vi "Move Picture Add Delta.vi"(6 "Delta":cluster{"y":i16, "x":i16}, 7 "Function":enum16{"nop", "point", "rect"}(ring), 9 "index":i32, 10 "Picture In":u8[](array[numeric])) -> (2 "Picture Out":u8[](array[numeric]))   [LabVIEW 2023]
doc: "Wiebe Walstra\nwww.carya.nl"
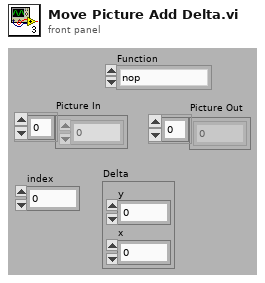
[diagram p1: front panel]
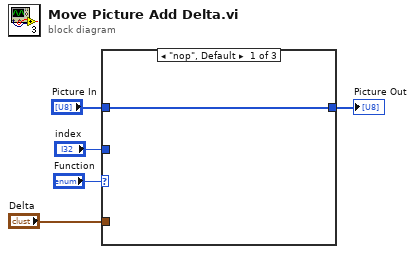
[diagram p0: block diagram]
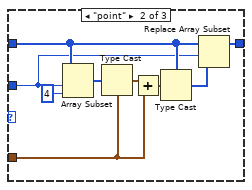
[diagram p2: hidden frame]
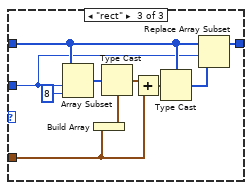
[diagram p3: hidden frame]
diagram:
  n1 = case shown="\"nop\", Default" "Function" {
    tunnel: [w6 w15 w25] -> w3
    tunnel: "Picture In" -> [w6 w10 w20]
    tunnel: "Delta" -> [_ w12 w22]
    tunnel: "index" -> [_ w8 w18]
    frame "nop", Default {
    }
    frame "point" {
      n2 = Array Subset(array=w10, index=w8, length=4) -> (w14:u8[])
      n3 = Type Cast(type=w12, x=w14) -> (*(type *) &x=w13:cluster{"y":i16, "x":i16})
      n4 = Add(x=w13, y=w12) -> (x+y=w11:cluster{"y":i16, "x":i16})
      n5 = Type Cast(type=w10, x=w11) -> (*(type *) &x=w9:u8[])
      n6 = Replace Array Subset(array=w10, new element=w9, index=w8) -> (w15:u8[])
    }
    frame "rect" {
      n7 = Array Subset(array=w20, index=w18, length=8) -> (w24:u8[])
      n8 = Build Array(w22) -> (w16:cluster{"y":i16, "x":i16}[])
      n9 = Type Cast(type=w16, x=w24) -> (*(type *) &x=w23:cluster{"y":i16, "x":i16}[])
      n10 = Add(x=w23, y=w22) -> (x+y=w21:cluster{"y":i16, "x":i16}[])
      n11 = Type Cast(type=w20, x=w21) -> (*(type *) &x=w19:u8[])
      n12 = Replace Array Subset(array=w20, new element=w19, index=w18) -> (w25:u8[])
    }
  }
  "Picture Out" <- w3
